vi "State History.vi"(7 "Current State":string, 11 "SMO":refnum<class "SMO.lvclass">) -> (3 "SMO out":refnum<class "SMO.lvclass">, 5 "History":string)   [LabVIEW 2019, in "Debug.lvlib"]
uses:
  Debug.lvlib
  <vilib>/JKI/JKI SMO/SMO/SMO.lvclass
  Attribute.Debug/DebugBehavior.ctl
  Attribute.Debug/Attribute.Debug.lvclass
panel:
  out "history length":i32=100
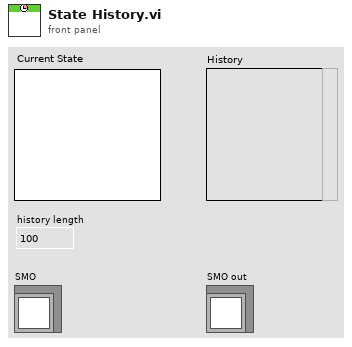
[diagram p1: front panel]
types:
  T1 = typedef "Debug.lvlib/Attribute.Debug.lvclass/DebugBehavior.ctl" = enum16{"Normal", "Debug"}
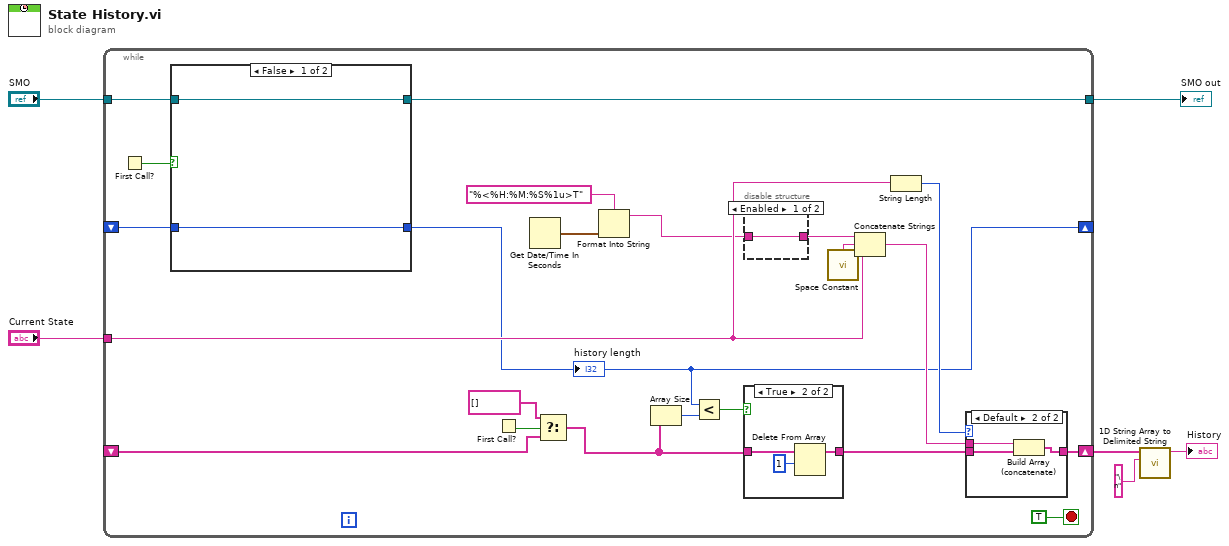
[diagram p0: block diagram]
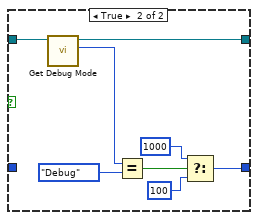
[diagram p2: hidden frame]
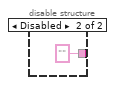
[diagram p3: hidden frame]
diagram:
  n1 = while {
    tunnel: "Current State" -> [w24]
    shift-right: [w25] -> w4
    shift-left: _ -> [w14]
    shift-right: [w7] -> _
    shift-left: _ -> [w8]
    tunnel: "SMO" -> [w11]
    tunnel: [w9] -> w1
    stop <- TRUE stop-if-true
    n2 = First Call?() -> (First Call?: T/F=w10:bool)
    n3 = case shown="False" w10 {
      tunnel: w11 -> [w30 w38]
      tunnel: [w30 w37] -> w9
      tunnel: [w29 w31] -> w7
      tunnel: w8 -> [w29 _]
      frame False {
      }
      frame True {
        n4 = call "Get Debug Mode.vi"("SMO"=w38) -> ("Behavior"=w35:T1, "SMO out"=w37:refnum<class "SMO.lvclass">)  [unwired: 8 in, 1 out]
        n5 = Equal?(x=w35, y=DebugBehavior."Debug" ("Behavior")) -> (x = y?=w34:bool)
        n6 = Select(t=1000 ("history length (100)"), s=w34, f=100 ("history length (100)")) -> (s? t:f=w31:i32)
      }
    }
    "history length" <- w7
    n7 = First Call?() -> (First Call?: T/F=w15:bool)
    n8 = Get Date/Time In Seconds() -> (seconds since 1Jan1904=w18:timestamp)
    n9 = Select(t=string[] [], s=w15, f=w14) -> (s? t:f=w13:string[])
    n10 = Format Into String(format string="%<%H:%M:%S%1u>T", w18) -> (resulting string=w16:string)  [unwired: 2 in, 1 out]
    n11 = Array Size(array=w13) -> (size(s)=w27:i32)
    n12 = Less?(x=w7, y=w27) -> (x < y?=w21:bool)
    n13 = case shown="True" w21 {
      tunnel: w13 -> [w45 w46]
      tunnel: [w45 w47] -> w28
      frame False {
      }
      frame True {
        n14 = Delete From Array(array=w46, length=1) -> (array with subset deleted=w47:string[])  [unwired: 1 in, 1 out]
      }
    }
    n15 = disable-structure shown="Enabled" {
      disable-tunnel: [w39 "" ("Spinner Out")] -> w23
      disable-tunnel: w16 -> [w39 _]
      frame Enabled {
      }
      frame Disabled {
      }
    }
    n16 = call <vilib>:"Space Constant.vi"() -> ("String"=w22:string)
    n17 = Concatenate Strings(w23, w22, w24) -> (w20:string)
    n18 = String Length(string=w24) -> (length=w19:i32)
    n19 = case shown="Default" w19 {
      tunnel: w28 -> [w41 w43]
      tunnel: [w41 w44] -> w25
      tunnel: w20 -> [_ w42]
      frame 0 {
      }
      frame Default {
        n20 = Build Array (concatenate)(w42, w43) -> (w44:string[])
      }
    }
  }
  "SMO out" <- w1
  n21 = call <vilib>:"1D String Array to Delimited String.vi"("delimiter"="\n", "string array"=w4) -> ("delimited string"=→"History":string)  [unwired: 9 in]
